vi "N330X_Measure_Voltage_Current.vi"() -> ()   [LabVIEW 2015]
panel:
  out "Maximum Voltage":dbl
  out "Minimum Voltage":dbl
  out "Total RMS Voltage":dbl
  out "Input Voltage":dbl
  out "error out":errorcluster
  out "VISA resource name out":refnum<visa-resource-name>
  out "Maximum Current":dbl
  out "Minimum Current":dbl
  out "Total RMS Current":dbl
  out "Input Current":dbl
  in  "error in (no error) 2":errorcluster
  in  "VISA resource name 2":refnum<visa-resource-name>
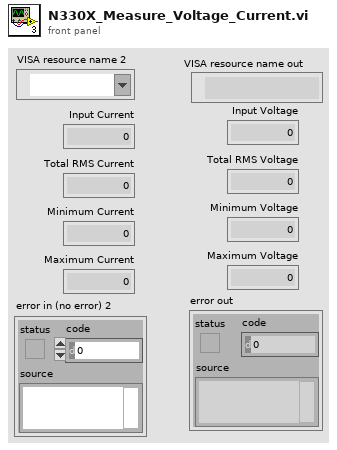
[diagram p1: front panel]
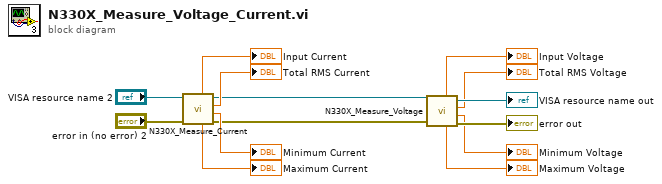
[diagram p0: block diagram]
diagram:
  n1 = call "N330X_Measure_Current.vi"("error in (no error)"="error in (no error) 2", "VISA Refnum in"="VISA resource name 2") -> ("error out"=w1:errorcluster, "Minimum Current"=→"Minimum Current":dbl, "Total RMS Current"=→"Total RMS Current":dbl, "VISA Refnum out"=w2:refnum<visa-resource-name>, "Maximum Current"=→"Maximum Current":dbl, "Input Current"=→"Input Current":dbl)  [unwired: 4 in]
  n2 = call "N330X_Measure_Voltage.vi"("error in (no error)"=w1, "VISA Refnum in"=w2) -> ("error out"=→"error out":errorcluster, "Minimum Voltage"=→"Minimum Voltage":dbl, "Total RMS Voltage"=→"Total RMS Voltage":dbl, "VISA Refnum out"=→"VISA resource name out":refnum<visa-resource-name>, "Maximum Voltage"=→"Maximum Voltage":dbl, "Input Voltage"=→"Input Voltage":dbl)  [unwired: 4 in]
